vi "ICM Simple Read Program(Scaling).vi"() -> ()   [LabVIEW 2018]
doc: "Test Program.vi\n\nThis is a simple program that uses the ICM to demonstrate its structure.\n\nInstrument Communication Module Version 1.0\nDecember, 2017 Original Code Consulting David Thomson\n www.originalcode.com"
uses:
  Scaling/Scaling.lvclass
  Scaling/Scaling.lvclass/Scaling.ctl
  Query/Query.lvclass/Query.ctl
  Query/Read Cycle Time (ms).vi
  Initialize/Initialize.lvclass
  Parser/Parser.lvclass
  Query/Query.lvclass
  Bus/Bus.lvclass
panel:
  out "Scaled Values":dbl[](array[numeric])
  in  "stop":bool
  out "Enabled Channels":string[](array[string])
  out "Data Values":dbl[](array[numeric])
  out "String Read":string
  out "error out":errorcluster
  out "Config File":path
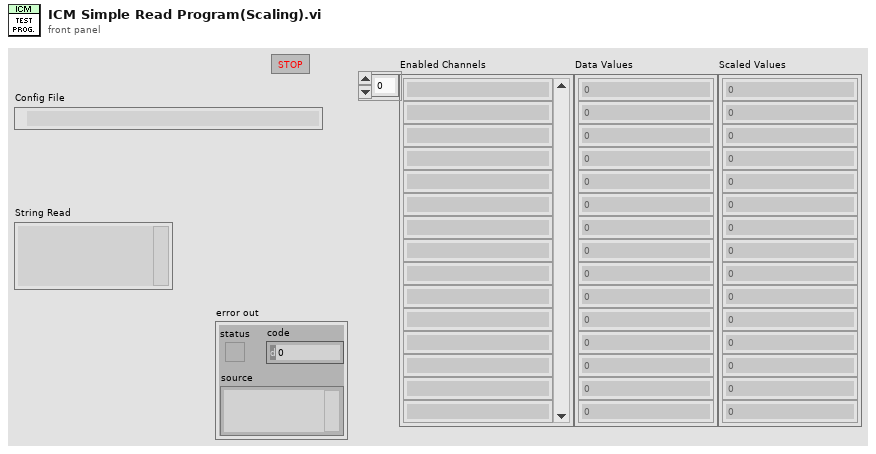
[diagram p1: front panel]
types:
  T1 = typedef "Scaling Def.ctl" = cluster{"Channel":string, "Scaling":string, "Instance":string}
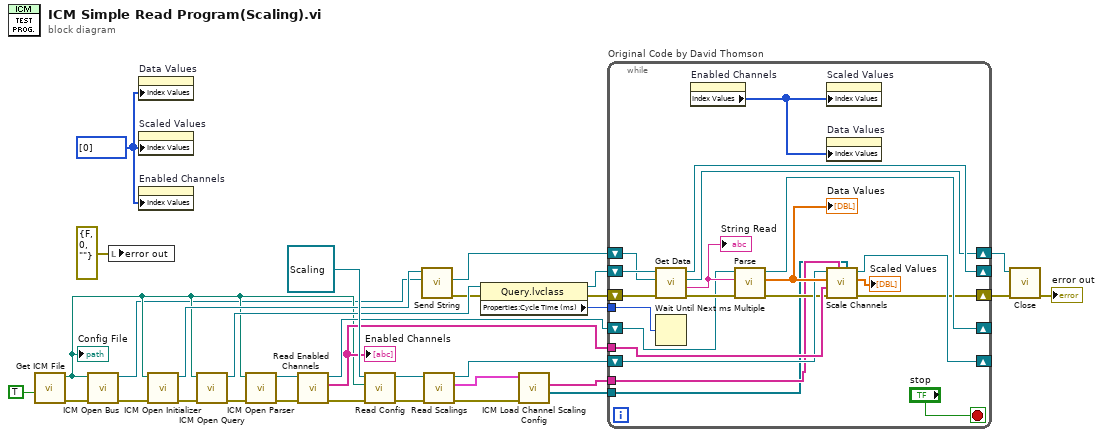
[diagram p0: block diagram]
diagram:
  w6 = u32[] [0] ("Index Values")
  n1 = call "Get ICM File.vi"("Re-Init?"=TRUE) -> ("error out"=w25:errorcluster, "ICM File"=w8:path)  [unwired: 9 in]
  "Config File" <- w8
  n2 = call "ICM Open Bus.vi"("error in (no error)"=w25, "ICM File In"=w8) -> ("error out"=w11:errorcluster, "Bus out"=w1:refnum<class "Bus.lvclass">)  [unwired: 8 in]
  n3 = local write "error out"(errorcluster {"status"=FALSE, "code"=0, "source"=""} ("error out")) -> ()
  n4 = property on="Data Values" class="Arr (strict)"("Index Values"=w6) -> ()  [unwired: 2 in, 2 out]
  n5 = property on="Scaled Values" class="Arr (strict)"("Index Values"=w6) -> ()  [unwired: 2 in, 2 out]
  n6 = property on="Enabled Channels" class="Arr (strict)"("Index Values"=w6) -> ()  [unwired: 2 in, 2 out]
  n7 = call "ICM Open Initializer.vi"("error in (no error)"=w11, "ICM File In"=w8) -> ("error out"=w7:errorcluster, "Init out"=w10:refnum<class "Initialize.lvclass">)  [unwired: 8 in]
  n8 = call "ICM Open Query.vi"("error in (no error)"=w7, "ICM File In"=w8) -> ("error out"=w26:errorcluster, "Query out"=w17:refnum<class "Query.lvclass">)  [unwired: 8 in]
  n9 = call "ICM Open Parser.vi"("error in (no error)"=w26, "ICM File In"=w8) -> ("error out"=w27:errorcluster, "Parser out"=w28:refnum<class "Parser.lvclass">)  [unwired: 8 in]
  n10 = call-dynamic "Read Enabled Channels.vi"("error in (no error)"=w27, "Parser in"=w28) -> ("error out"=w24:errorcluster, "Enabled Channels"=w22:string[], "Parser out"=w12:refnum<class "Parser.lvclass">)  [unwired: 7 in]
  "Enabled Channels" <- w22
  n11 = call-dynamic "Read Config.vi"("error in (no error)"=w24, "ICM File In"=w8, "Scaling in"=refnum<class "Scaling.lvclass"> refnum) -> ("error out"=w21:errorcluster, "Scaling out"=w19:refnum<class "Scaling.lvclass">)  [unwired: 7 in]
  n12 = call-dynamic "Send String.vi"("Bus In"=w1, "Init in"=w10) -> ("error out"=w9:errorcluster, "Bus Out"=w2:refnum<class "Bus.lvclass">)  [unwired: 5 in, 1 out]
  n13 = call "Read Scalings.vi"("error in (no error)"=w21, "Scaling in"=w19) -> ("error out"=w20:errorcluster, "Scalings"=w18:T1[], "Scaling out"=w4:refnum<class "Scaling.lvclass">)  [unwired: 7 in]
  n14 = property class="Query.lvclass"(reference=w17, error in=w9) -> (reference out=w16:refnum<class "Query.lvclass">, error out=w14:errorcluster, "Properties:Cycle Time (ms)"=w15:u32)
  n15 = call "ICM Load Channel Scaling Config.vi"("error in (no error)"=w20, "Scalings"=w18) -> ("Scaling Classes"=w5:refnum<class "Scaling.lvclass">[], "Used Scalings"=w3:string[])  [unwired: 6 in, 2 out]
  n16 = while "Original Code by David Thomson" {
    shift-right: [w33] -> w30
    shift-left: w14 -> [w51]
    tunnel: w15 -> [w49]
    tunnel: w22 -> [w46]
    tunnel: w3 -> [w37]
    tunnel: w5 -> [w36]
    shift-right: [w34] -> w31
    shift-left: w2 -> [w48]
    shift-right: [w43] -> _
    shift-left: w12 -> [w44]
    shift-right: [w42] -> _
    shift-left: w16 -> [w52]
    shift-right: [w38] -> _
    shift-left: w4 -> [w41]
    stop <- "stop" stop-if-true
    n17 = call-dynamic "Get Data.vi"("error in (no error)"=w51, "Bus In"=w48, "Query in"=w52) -> ("error out"=w50:errorcluster, "String Read"=w53:string, "Bus Out"=w34:refnum<class "Bus.lvclass">, "Query out"=w42:refnum<class "Query.lvclass">)  [unwired: 5 in]
    "String Read" <- w53
    n18 = Wait Until Next ms Multiple(millisecond multiple=w49) -> ()  [unwired: 1 out]
    n19 = property on="Enabled Channels" class="Arr (strict)"() -> ("Index Values"=w39:u32[])  [unwired: 2 in, 2 out]
    n20 = call-dynamic "Parse.vi"("error in (no error)"=w50, "Data String"=w53, "Parser in"=w44) -> ("error out"=w40:errorcluster, "Data Values"=w47:dbl[], "Parser out"=w43:refnum<class "Parser.lvclass">)  [unwired: 6 in]
    "Data Values" <- w47
    n21 = property on="Scaled Values" class="Arr (strict)"("Index Values"=w39) -> ()  [unwired: 2 in, 2 out]
    n22 = property on="Data Values" class="Arr (strict)"("Index Values"=w39) -> ()  [unwired: 2 in, 2 out]
    n23 = call "Scale Channels.vi"("Scaling Classes"=w36, "Used Scalings"=w37, "error in (no error)"=w40, "Channel Names"=w46, "Values In"=w47, "Scaling in"=w41) -> ("error out"=w33:errorcluster, "Values Out"=→"Scaled Values":dbl[], "Scaling out"=w38:refnum<class "Scaling.lvclass">)  [unwired: 3 in]
  }
  n24 = call-dynamic "Close.vi"("error in (no error)"=w30, "Bus in"=w31) -> ("error out"=→"error out":errorcluster)  [unwired: 8 in, 1 out]
